vi "MS Operation v2.vi"(6 "PID Cluster":T3={"L1 to L4 PID Cluster"={"L1 PID Gains"={"Kp"=0.005, "Kd"=0.5, "Ki"=0.0005}, "L2 PID Gains"={"Kp"=0.01, "Kd"=1.0, "Ki"=0.005}, "L3 PID Gains"={"Kp"=0.05, "Kd"=1.0, "Ki"=0.0005}, "L4 PID Gains"={"Kp"=0.1, "Kd"=0.1, "Ki"=0.0005}}, "Stage PID Cluster"={"Stage Z PID"={"Kp"=0.0005, "Kd"=0.001, "Ki"=0.0}, "Stage Y PID"={"Kp"=0.0003, "Kd"=0.01, "Ki"=0.0}, "Stage X PID"={"Kp"=0.0003, "Kd"=0.01, "Ki"=0.0}}, "OCT Z PID Gains"={"Kp"=0.0003, "Kd"=0.0001, "Ki"=0.01}}, 7 "Robot In":i32, 8 "error in":errorcluster, 10 "Prev Posit Cluster":T2={"Prev L1 to L4 Posit"=[-0.5319, -0.035669172703475985, -2.0566170657346783, 0.9099264705882353], "Prev Stage Posit"=[6.002553885707208, 5.996566124542428, 5.995469940427586], "Prev OCT Z Posit"=-0.0}, 11 "FPGA VI Reference In":refnum<k20>) -> (0 "error out":errorcluster, 2 "Last Posit Cluster":T1={"Last L1 to L4 Posit"=[0.0, 0.0, 0.0, 0.0], "Last Stage Posit"=[6.0, 6.0, 6.0], "Last OCT Z Posit"=0.0}, 3 "FPGA VI Reference Out":refnum<k20>)   [LabVIEW 2016]
uses:
  Subsystems/Global Variables.vi
  <vilib>/Platform/TimedLoop/XDataNode/wakeup.ctl
  <vilib>/Platform/TimedLoop/XDataNode/XDNodeRunTimeDep.lvlib
  <vilib>/Platform/TimedLoop/XDataNode/nitl_modes.ctl
  <vilib>/Platform/TimedLoop/XDataNode/timing_clust.ctl
  <vilib>/platform/TimedLoop/XDataNode/XDataNode.xnode
  <vilib>/rvi/interface/nirviReadWriteControl/nirviReadWriteControl.xnode
  Library/KevinLibraryAll/labview/KevLib01.lvlib
  FPGA Bitfiles/PhantomControlPI_FPGATarget_QuadCtr2_E2412E44.lvbitx
  IRISS_FPGA_IO.vi
  NiFpgaLv.dll
  <vilib>/Utility/error.llb/Error Cluster From Error Code.vi
  <vilib>/rvi/errors/niLvFpgaAdjustHostInterfaceError.vi
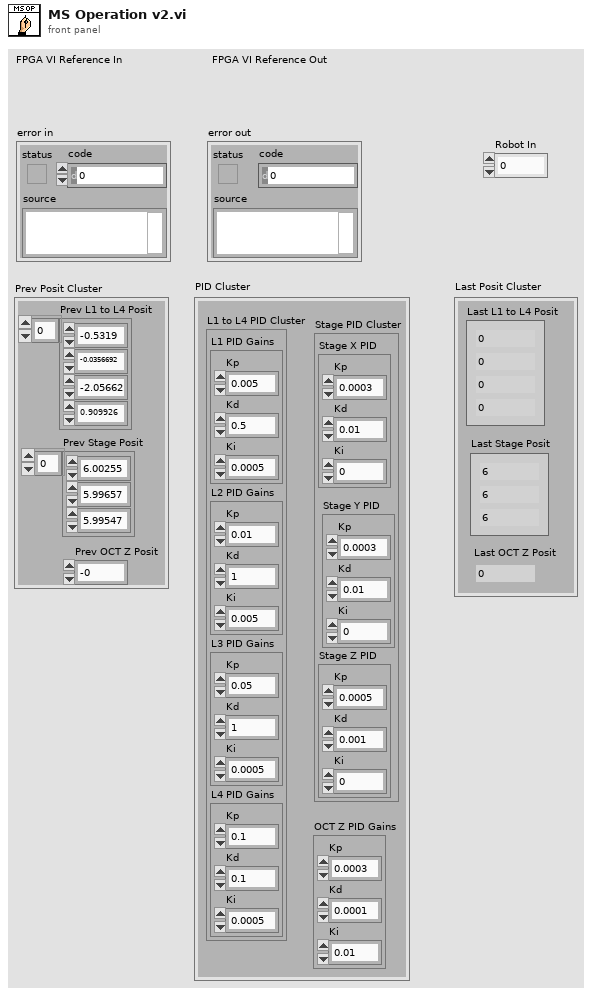
[diagram p1: front panel]
types:
  T1 = cluster{"Last L1 to L4 Posit":dbl[], "Last Stage Posit":dbl[], "Last OCT Z Posit":dbl}
  T2 = cluster{"Prev L1 to L4 Posit":dbl[], "Prev Stage Posit":dbl[], "Prev OCT Z Posit":dbl}
  T3 = cluster{"L1 to L4 PID Cluster":cluster{"L1 PID Gains":cluster{"Kp":dbl, "Kd":dbl, "Ki":dbl}, "L2 PID Gains":cluster{"Kp":dbl, "Kd":dbl, "Ki":dbl}, "L3 PID Gains":cluster{"Kp":dbl, "Kd":dbl, "Ki":dbl}, "L4 PID Gains":cluster{"Kp":dbl, "Kd":dbl, "Ki":dbl}}, "Stage PID Cluster":cluster{"Stage Z PID":cluster{"Kp":dbl, "Kd":dbl, "Ki":dbl}, "Stage Y PID":cluster{"Kp":dbl, "Kd":dbl, "Ki":dbl}, "Stage X PID":cluster{"Kp":dbl, "Kd":dbl, "Ki":dbl}}, "OCT Z PID Gains":cluster{"Kp":dbl, "Kd":dbl, "Ki":dbl}}
  T4 = typedef "XDNodeRunTimeDep.lvlib/timing_clust.ctl" = cluster{"Expected End [f-1]":u64, "Actual End [f-1]":u64, "Finished Late? [f-1]":bool, "Expected End [i-1]":u64, "Actual End [i-1]":u64, "Finished Late? [i-1]":bool, "Expected Start [i]":u64, "Actual Start [i]":u64, "Expected Start [f]":u64, "Actual Start [f]":u64, "Source Name":string, "Structure Name":string, "Period":i64, "Deadline":i64, "Offset":i64, "Start":i64, "Priority":i32, "Timeout":i32, "Mode":T5, "Wakeup Reason":T6, "Error":errorcluster, "Source Type":string, "Secondary Source Type":string, "Global End Time":u64, "Global Start Time":u64, "Frame Duration":u64, "Iteration Duration":u64, "Assigned CPU":i32, "I/O Scan Engine Mode":u32}
  T5 = typedef "XDNodeRunTimeDep.lvlib/nitl_modes.ctl" = enum32{"No Change", "Process missed periods, maintain original phase", "Discard missed periods, maintain original phase", "Process missed periods, ignore original phase", "Discard missed periods, ignore original phase"}
  T6 = typedef "XDNodeRunTimeDep.lvlib/wakeup.ctl" = enum32{"Normal", "Aborted", "Asynchronous wakeup", "Timing source error", "Timed loop error", "Timeout"}
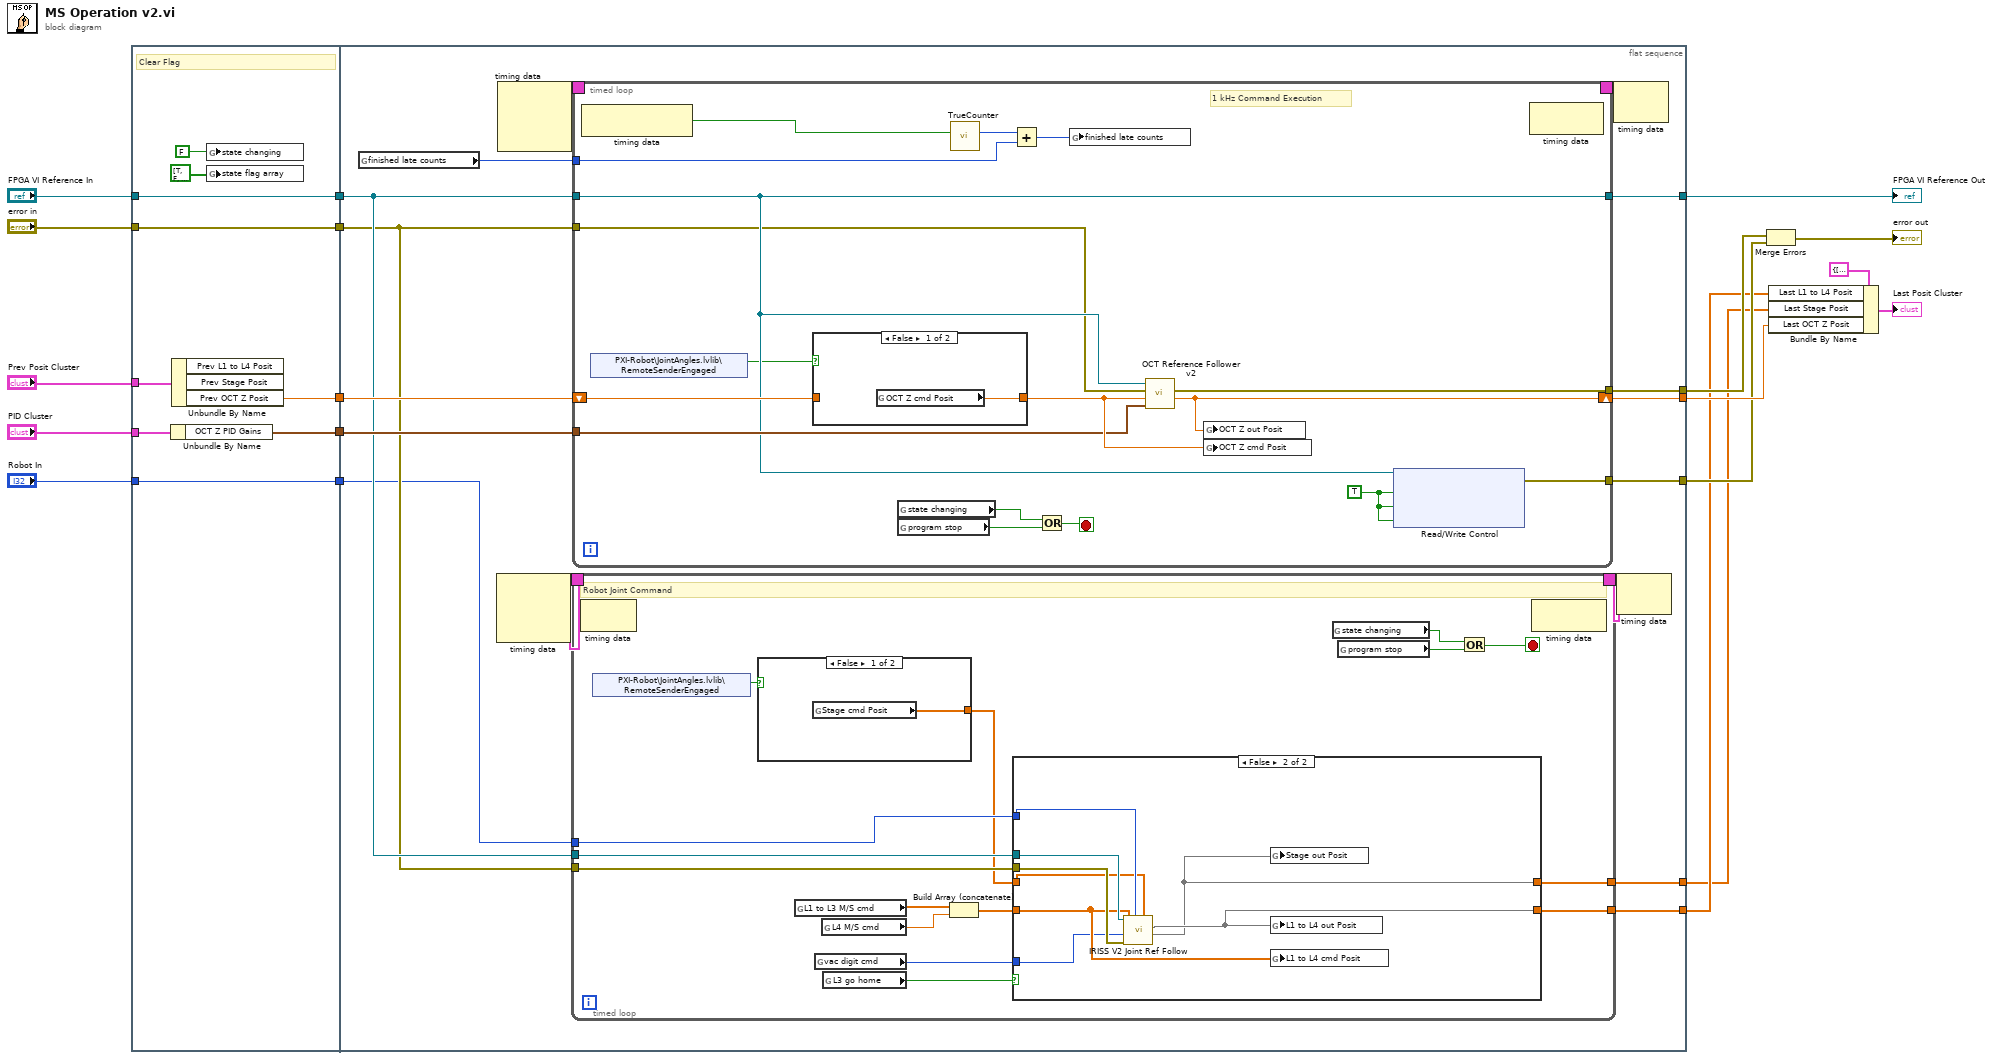
[diagram p0: block diagram]
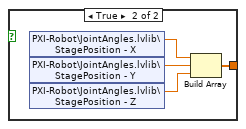
[diagram p2: hidden frame]
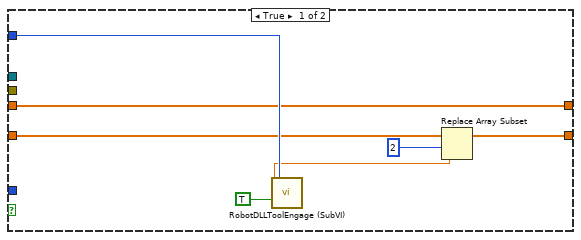
[diagram p3: hidden frame]
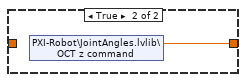
[diagram p4: hidden frame]
diagram:
  n1 = flat-sequence {
    tunnel: [w26] -> w19
    tunnel: "FPGA VI Reference In" -> [w26]
    tunnel: [w25] -> w17
    tunnel: "error in" -> [w25]
    tunnel: "Prev Posit Cluster" -> [w22]
    tunnel: "PID Cluster" -> [w24]
    tunnel: [w23] -> w10
    tunnel: [w21] -> w9
    tunnel: "Robot In" -> [w20]
    tunnel: [w20] -> w3
    tunnel: w19 -> [w34]
    tunnel: w17 -> [w33]
    tunnel: [w40] -> w6
    tunnel: [w39] -> w7
    tunnel: [w35] -> w11
    tunnel: w10 -> [w38]
    tunnel: w9 -> [w36]
    tunnel: [w32] -> w5
    tunnel: w3 -> [w30]
    tunnel: [w31] -> w2
    tunnel: [w29] -> w1
    frame #0 {
      # "Clear Flag"
      n2 = Unbundle By Name(w24) -> ("OCT Z PID Gains"=w23:cluster{"Kp":dbl, "Kd":dbl, "Ki":dbl})
      n3 = Unbundle By Name(w22) -> ("Prev OCT Z Posit"=w21:dbl)  [unwired: 2 out]
      n4 = global write "Global Variables.vi" "state changing"(FALSE ("state changing")) -> ()
      n5 = global write "Global Variables.vi" "state flag array"(bool[] [TRUE, FALSE, FALSE, FALSE, FALSE, FALSE, FALSE, FALSE, FALSE] ("state flag array")) -> ()
    }
    frame #1 {
      n6 = global read "Global Variables.vi" "finished late counts"() -> (w37:u16)
      n7 = node-c288() -> (w42:T4)  [unwired: 3 in]
      n8 = node-c288() -> (w44:T4)  [unwired: 3 in]
      n9 = timed-loop {
        timing: w42 -> [_]
        timing-out: [_] -> w41
        tunnel: w34 -> [w53]
        tunnel: w33 -> [w52]
        tunnel: [w55] -> w32
        tunnel: w30 -> [w54]
        tunnel: [w46] -> w29
        stop <- w59 stop-if-true
        # "Robot Joint Command"
        n10 = node-c288() -> ()  [unwired: 1 in, 1 out]
        n11 = shared-variable "PXI-Robot\\JointAngles.lvlib\\RemoteSenderEngaged"() -> (w47:bool)  [unwired: 1 in, 1 out]
        n12 = case shown="False" w47 {
          tunnel: [w60 w64] -> w45
          frame False {
            n13 = global read "Global Variables.vi" "Stage cmd Posit"() -> (w60:dbl[])
          }
          frame True {
            n14 = shared-variable "PXI-Robot\\JointAngles.lvlib\\StagePosition - X"() -> (w61:dbl)  [unwired: 1 in, 1 out]
            n15 = shared-variable "PXI-Robot\\JointAngles.lvlib\\StagePosition - Y"() -> (w62:dbl)  [unwired: 1 in, 1 out]
            n16 = shared-variable "PXI-Robot\\JointAngles.lvlib\\StagePosition - Z"() -> (w63:dbl)  [unwired: 1 in, 1 out]
            n17 = Build Array(w61, w62, w63) -> (w64:dbl[])
          }
        }
        n18 = global read "Global Variables.vi" "L1 to L3 M/S cmd"() -> (w48:dbl[])
        n19 = global read "Global Variables.vi" "vac digit cmd"() -> (w51:i8)
        n20 = global read "Global Variables.vi" "L4 M/S cmd"() -> (w50:dbl)
        n21 = global read "Global Variables.vi" "L3 go home"() -> (w56:bool)
        n22 = Build Array (concatenate)(w48, w50) -> (w49:dbl[])
        n23 = case shown="False" w56 {
          tunnel: w54 -> [w70 w75]
          tunnel: w53 -> [_ w79]
          tunnel: w52 -> [_ w78]
          tunnel: w49 -> [w66 w77]
          tunnel: [w67 w74] -> w55
          tunnel: w51 -> [_ w76]
          tunnel: w45 -> [w65 w73]
          tunnel: [w65 w72] -> w46
          frame True {
            n24 = call "RobotDLLToolEngage (SubVI).vi"("Tool Fast Retraction"=TRUE ("Tool Withdraw"), "ArmID"=w70) -> ("actInsertionLength"=w68:dbl)  [unwired: 17 in]
            n25 = Replace Array Subset(array=w66, new element=w68, index=2) -> (w67:dbl[])
          }
          frame False {
            n26 = call "IRISS V2 Joint Ref Follow.vi"(4:w73, 5:w75, "error in"=w78, "Digital Cmd [0-78]"=w76, 8:w77, "FPGA VI Reference In"=w79) -> (1:w72, 2:w74)  [unwired: 2 out]
            n27 = global write "Global Variables.vi" "Stage out Posit"(w72) -> ()
            n28 = global write "Global Variables.vi" "L1 to L4 out Posit"(w74) -> ()
            n29 = global write "Global Variables.vi" "L1 to L4 cmd Posit"(w77) -> ()
          }
        }
        n30 = global read "Global Variables.vi" "state changing"() -> (w58:bool)
        n31 = global read "Global Variables.vi" "program stop"() -> (w57:bool)
        n32 = Or(x=w58, y=w57) -> (x .or. y?=w59:bool)
        n33 = node-c288() -> ()  [unwired: 1 in, 1 out]
      }
      n34 = timed-loop {
        timing: w44 -> [_]
        timing-out: [_] -> w43
        tunnel: w34 -> [w87]
        tunnel: w33 -> [w86]
        tunnel: [w98] -> w40
        tunnel: [w87] -> w31
        tunnel: [w89] -> w39
        tunnel: w38 -> [w90]
        tunnel: w37 -> [w93]
        shift-right: [w88] -> w35
        shift-left: w36 -> [w92]
        stop <- w100 stop-if-true
        w84 = TRUE ("Conn0/DIO15 Button 4")
        # "1 kHz Command Execution"
        n35 = node-c288() -> (w96:bool)  [unwired: 1 in]
        n36 = shared-variable "PXI-Robot\\JointAngles.lvlib\\RemoteSenderEngaged"() -> (w85:bool)  [unwired: 1 in, 1 out]
        n37 = case shown="False" w85 {
          tunnel: [w101 w102] -> w91
          tunnel: w92 -> [_ _]
          frame False {
            n38 = global read "Global Variables.vi" "OCT Z cmd Posit"() -> (w101:dbl)
          }
          frame True {
            n39 = shared-variable "PXI-Robot\\JointAngles.lvlib\\OCT z command"() -> (w102:dbl)  [unwired: 1 in, 1 out]
          }
        }
        n40 = global read "Global Variables.vi" "state changing"() -> (w99:bool)
        n41 = global read "Global Variables.vi" "program stop"() -> (w97:bool)
        n42 = call "TrueCounter.vi"("True?"=w96) -> ("True Count"=w94:u16)  [unwired: 10 in]
        n43 = Add(x=w94, y=w93) -> (x+y=w95:u16)
        n44 = Or(x=w99, y=w97) -> (x .or. y?=w100:bool)
        n45 = global write "Global Variables.vi" "finished late counts"(w95) -> ()
        n46 = call "OCT Reference Follower v2.vi"("OCT Z PID Gains"=w90, "OCT  Z cmd Posit [mm]"=w91, "error in"=w86, "FPGA VI Reference In"=w87) -> ("OCT  Z out Posit [mm]"=w88:dbl, "error out"=w89:errorcluster)  [unwired: 5 in, 1 out]
        n47 = global write "Global Variables.vi" "OCT Z out Posit"(w88) -> ()
        n48 = global write "Global Variables.vi" "OCT Z cmd Posit"(w91) -> ()
        n49 = xnode "Read/Write Control"("FPGA VI Reference In"=w87, "Conn0/DIO12 Button 1"=w84, "Conn0/DIO13 Button 2"=w84, "Conn0/DIO15 Button 4"=w84) -> ("error out"=w98:errorcluster)  [unwired: 1 in, 1 out]
        n50 = node-c288() -> ()  [unwired: 1 in, 1 out]
      }
      n51 = node-c288(w43) -> ()  [unwired: 1 out]
      n52 = node-c288(w41) -> ()  [unwired: 1 out]
    }
  }
  n53 = Merge Errors(w7, w6) -> (→"error out":errorcluster)
  n54 = Bundle By Name(cluster=T1 {"Last L1 to L4 Posit"=[-0.5607, -0.038216970753724266, -2.0806193533568895, 1.1787683823529411], "Last Stage Posit"=[6.002553885707208, 5.996566124542428, 5.995469940427586], "Last OCT Z Posit"=-0.0} ("Last Posit Cluster 2"), "Last L1 to L4 Posit"=w5, "Last Stage Posit"=w1, "Last OCT Z Posit"=w11) -> (→"Last Posit Cluster":T1)
  "FPGA VI Reference Out" <- w2
